vi "lab2_3.vi"() -> ()   [LabVIEW 2017]
panel:
  out "reszta":dbl
  out "wynik dzielenia":dbl
  in  "liczba2":dbl
  in  "liczba1":dbl
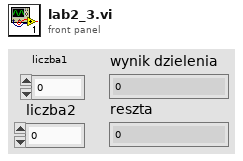
[diagram p1: front panel]
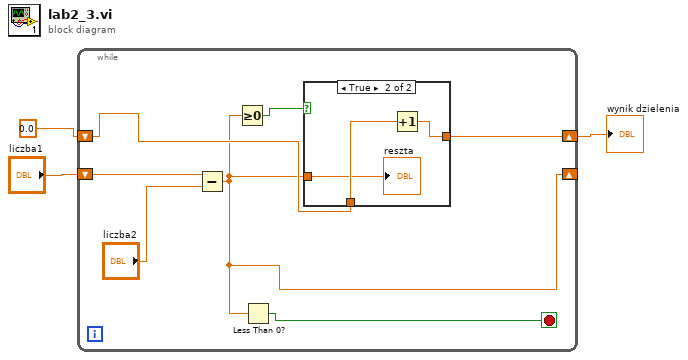
[diagram p0: block diagram]
diagram:
  n1 = while {
    shift-right: [w10] -> w3
    shift-left: 0.0 ("wynik dzielenia") -> [w5]
    shift-right: [w4] -> _
    shift-left: "liczba1" -> [w6]
    stop <- w8 stop-if-true
    n2 = Subtract(x=w6, y="liczba2") -> (x-y=w4:dbl)
    n3 = Greater Or Equal To 0?(x=w4) -> (x >= 0?=w9:bool)
    n4 = Less Than 0?(x=w4) -> (x < 0?=w8:bool)
    n5 = case shown="True" w9 {
      tunnel: w5 -> [w11 w14]
      tunnel: [w11 w13] -> w10
      tunnel: w4 -> [_ w12]
      frame False {
      }
      frame True {
        n6 = Increment(x=w14) -> (x+1=w13:dbl)
        "reszta" <- w12
      }
    }
  }
  "wynik dzielenia" <- w3
